vi "DDGImage_.VI"() -> ()   [LabVIEW 2012]
uses:
  <userlib>/atmcd32d.llb/Spool_method typedef.ctl
panel:
  in  "array":i32[](array[numeric])
  out "err string 2":string
  out "强度图 2":i32[][](graph)
  out "err string":string
  out "error out 2":errorcluster
  out "error out":errorcluster
  out "last":i32
  out "first":u32
  out "布尔":bool
  out "强度图":i32[][](graph)
  out "Calculated Kinetic Cycle Time":sgl format="%.2f"
  in  "Frequency (Hz):":dbl format="%.2f"
  in  "Integrate on chip":bool
  in  "Gate step (nsecs)":i32 step=25
  in  "Pulse Width (nsecs)":i32=1000
  in  "Delay (nsecs)":i32 step=25
  in  "Output A Delay (nsecs)":i32 min=0 step=16
  in  "Gain (0-255)":i32 min=0 max=255
  in  "Kinetic Cycle Time":sgl format="%.2f"
  in  "Shut Down":bool
  in  "Start Acquisition":bool
  out "Return  from Get Acquired Data":u32
  out "Detector X Pixels":i32
  out "Return from GetStatus":u32
  out "Return from Start Acquisition":u32
  in  "Number of Kinetics":i32=5
  out "Return from CheckTimings Exposure":u32
  out "Calculated Exposure Value":sgl format="%.2f"
  in  "Exposure Time (secs)":sgl=0.05 format="%.2f"
  out "Return from Initialize":u32
  in  "Trigger":u32(ring) items=["Internal", "External"]
  # "Acquisition Mode: Kinetics\nReadout Mode: Full Image.  Only showing one image of data."
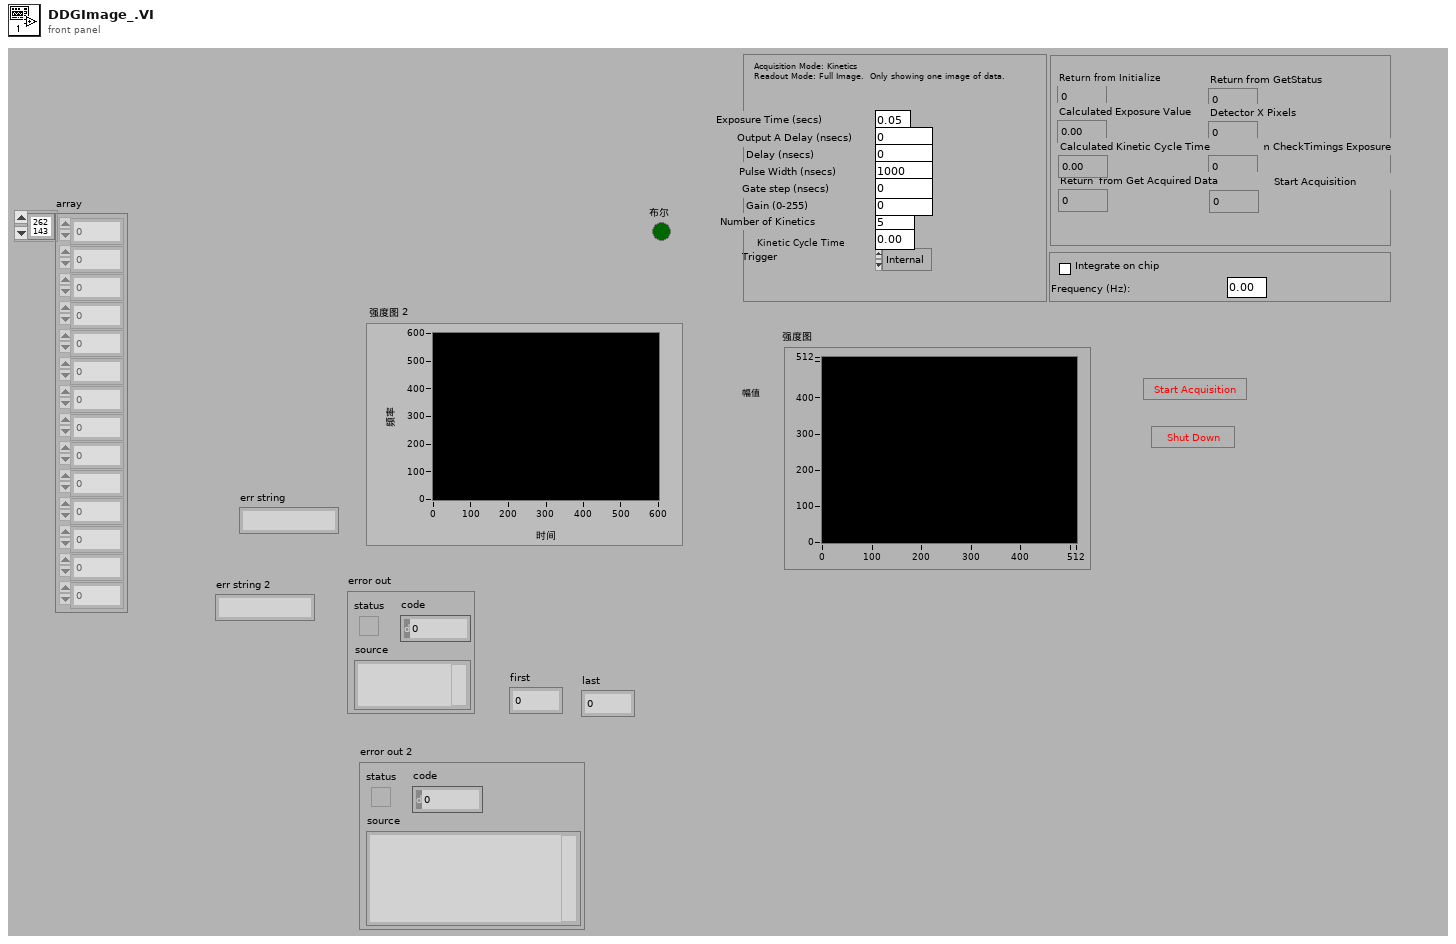
[diagram p1: front panel]
types:
  T1 = typedef "Spool_method typedef.ctl" = enum16{"32-bit", "Depends", "16-bit", "Multiple Directory", "Spool to RAM disk", "16-bit FITS", "SIF", "16-buit TIFF", "Multiple Directory Compressed"}
  T2 = typedef "Error Code Enum typedef.ctl" = enum32{"N/A (0)", "DRV_ERROR_CODES", "DRV_SUCCESS", "DRV_VXDNOTINSTALLED", "DRV_ERROR_SCAN", "DRV_ERROR_CHECK_SUM", "DRV_ERROR_FILELOAD", "DRV_UNKNOWN_FUNC", "DRV_ERROR_VXD_INIT", "DRV_ERROR_ADDRESS", "DRV_ERROR_PAGELOCK", "DRV_ERROR_PAGEUNLOCK", "DRV_ERROR_BOARDTEST", "DRV_ERROR_ACK", "DRV_ERROR_UP_FIFO", "DRV_ERROR_PATTERN", "N/A (16)", "DRV_ACQUISITION_ERRORS", "DRV_ACQ_BUFFER", "DRV_ACQ_DOWNFIFO_FULL", "DRV_PROC_UNKONWN_INSTRUCTION", "DRV_ILLEGAL_OP_CODE", "DRV_KINETIC_TIME_NOT_MET", "DRV_ACCUM_TIME_NOT_MET", "DRV_NO_NEW_DATA", "N/A (25)", "DRV_SPOOLERROR", "N/A (27)", "N/A (28)", "N/A (29)", "N/A (30)", "N/A (31)", "N/A (32)", "DRV_TEMPERATURE_CODES", "DRV_TEMPERATURE_OFF", "DRV_TEMPERATURE_NOT_STABILIZED", "DRV_TEMPERATURE_STABILIZED", "DRV_TEMPERATURE_NOT_REACHED", "DRV_TEMPERATURE_OUT_RANGE", "DRV_TEMPERATURE_NOT_SUPPORTED", "DRV_TEMPERATURE_DRIFT", "N/A (41)", "N/A (42)", "N/A (43)", "N/A (44)", "N/A (45)", "N/A (46)", "N/A (47)", "N/A (48)", "DRV_GENERAL_ERRORS", "DRV_INVALID_AUX", "DRV_COF_NOTLOADED", "DRV_FPGAPROG", "DRV_FLEXERROR", "DRV_GPIBERROR", "N/A (55)", "N/A (56)", "N/A (57)", "N/A (58)", "N/A (59)", "N/A (60)", "N/A (61)", "N/A (62)", "N/A (63)", "DRV_DATATYPE", "DRV_DRIVER_ERRORS", "DRV_P1INVALID", "DRV_P2INVALID", "DRV_P3INVALID", "DRV_P4INVALID", "DRV_INIERROR", "DRV_COFERROR", "DRV_ACQUIRING", "DRV_IDLE", "DRV_TEMPCYCLE", "DRV_NOT_INITIALIZED", "DRV_P5INVALID", "DRV_P6INVALID", "DRV_INVALID_MODE", "DRV_INVALID_FILTER", "DRV_I2CERRORS", "DRV_I2CDEVNOTFOUND", "DRV_I2CTIMEOUT", "DRV_P7INVALID", "N/A (84)", "N/A (85)", "N/A (86)", "N/A (87)", "N/A (88)", "N/A (89)", "DRV_IOCERROR", "DRV_VRMVERSIONERROR"}
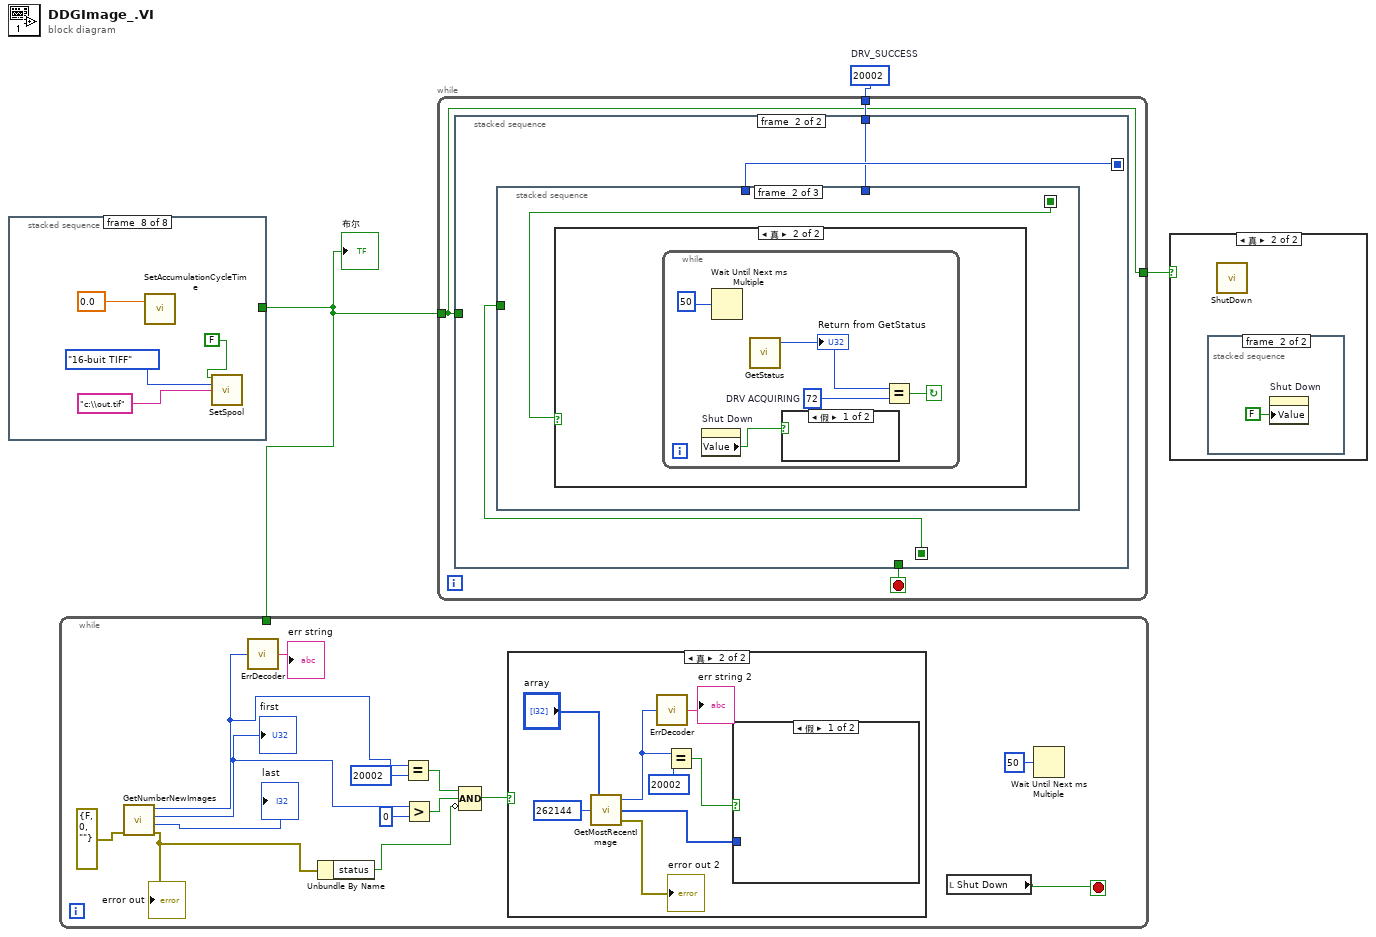
[diagram p0: block diagram]
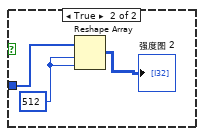
[diagram p3: hidden frame]
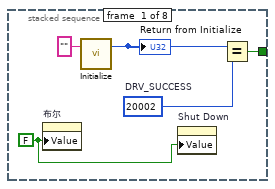
[diagram p4: hidden frame]
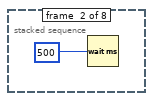
[diagram p5: hidden frame]
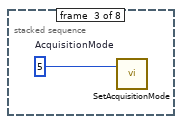
[diagram p6: hidden frame]
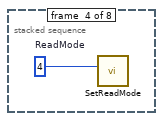
[diagram p7: hidden frame]
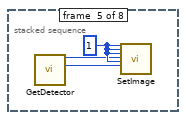
[diagram p8: hidden frame]
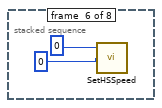
[diagram p9: hidden frame]
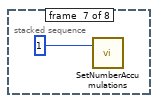
[diagram p10: hidden frame]
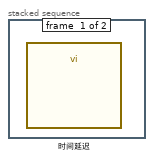
[diagram p12: hidden frame]
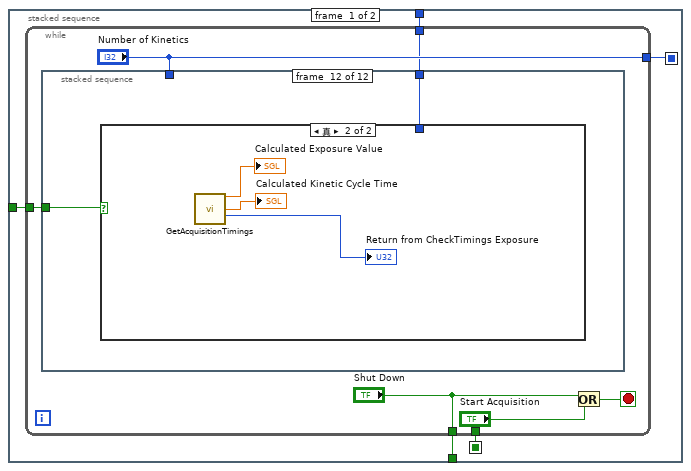
[diagram p13: hidden frame]
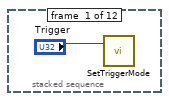
[diagram p14: hidden frame]
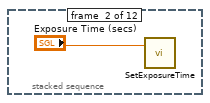
[diagram p15: hidden frame]
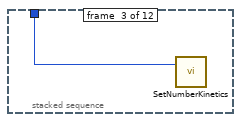
[diagram p16: hidden frame]
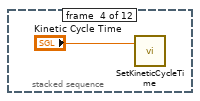
[diagram p17: hidden frame]
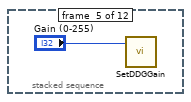
[diagram p18: hidden frame]
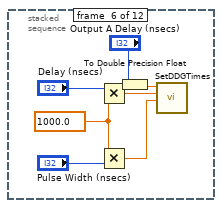
[diagram p19: hidden frame]
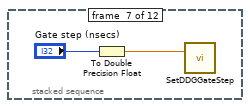
[diagram p20: hidden frame]
diagram:
  w2 = 20002  # DRV_SUCCESS
  n1 = stacked-sequence {
    tunnel: [w5 _ _ _ _ _ _ _] -> w1
    frame #0 {
      w4 = FALSE ("布尔")
      w6 = 20002  # DRV_SUCCESS
      n2 = property on="布尔" class="Bool (严格)"("Value"=w4) -> ()  [unwired: 2 in, 2 out]
      n3 = call <userlib>:"Initialize.vi"("directory (\"\")"="" ("directory (\"\")")) -> ("DLL error code"=w7:u32)  [unwired: 1 in, 1 out]
      "Return from Initialize" <- w7
      n4 = property on="Shut Down" class="Bool (严格)"("Value"=w4) -> ()  [unwired: 2 in, 2 out]
      n5 = Equal?(x=w7, y=w6) -> (x = y?=w5:bool)
    }
    frame #1 {
      n6 = Wait (ms)(milliseconds to wait=u32 500) -> ()  [unwired: 1 out]
    }
    frame #2 {
      w10 = u16 5  # AcquisitionMode
      n7 = call <userlib>:"SetAcquisitionMode.vi"("mode"=w10) -> ()  [unwired: 1 in, 2 out]
    }
    frame #3 {
      w11 = u16 4  # ReadMode
      n8 = call <userlib>:"SetReadMode.vi"("mode"=w11) -> ()  [unwired: 1 in, 2 out]
    }
    frame #4 {
      w14 = 1
      n9 = call <userlib>:"GetDetector.vi"() -> ("ypixels"=w12:i32, "xpixels"=w13:i32)  [unwired: 4 in, 2 out]
      n10 = call <userlib>:"SetImage.vi"("hbin"=w14, "vbin"=w14, "hstart"=w14, "hend"=w13, "vstart"=w14, "vend"=w12) -> ()  [unwired: 20 in, 2 out]
    }
    frame #5 {
      n11 = call <userlib>:"SetHSSpeed.vi"("index"=0, "type"=0) -> ()  [unwired: 2 in, 2 out]
    }
    frame #6 {
      n12 = call <userlib>:"SetNumberAccumulations.vi"("number"=1) -> ()  [unwired: 1 in, 2 out]
    }
    frame #7 {
      n13 = call <userlib>:"SetAccumulationCycleTime.vi"("time"=sgl 0.0) -> ()  [unwired: 1 in, 2 out]
      n14 = call <userlib>:"SetSpool.vi"("active"=FALSE, "method"=Spool_method_typedef."16-buit TIFF", "name"="c:\\out.tif") -> ()  [unwired: 11 in, 2 out]
    }
  }
  "布尔" <- w1
  n15 = while {
    tunnel: w1 -> [_]
    stop <- w24 stop-if-true
    n16 = call <userlib>:"GetNumberNewImages.vi"("error in (no error)"=errorcluster {"status"=FALSE, "code"=0, "source"=""}) -> ("error out"=w32:errorcluster, "last"=→"last":i32, "first"=w30:u32, "DLL error code"=w23:u32)  [unwired: 3 in]
    "first" <- w30
    "error out" <- w32
    n17 = call "ErrDecoder.vi"("err code"=w23) -> ("err string"=→"err string":string)
    n18 = Unbundle By Name(w32) -> ("status"=w26:bool)
    n19 = Equal?(x=w23, y=u32 20002) -> (x = y?=w28:bool)
    n20 = Greater?(x=w30, y=u32 0) -> (0:w27:bool)
    n21 = Compound Arithmetic op=AND(w28, w27, invert w26) -> (w25:bool)
    n22 = case shown="真" w25 {
      frame False {
      }
      frame True {
        n23 = call <userlib>:"GetMostRecentImage.vi"("size"=262144, "array"="array") -> ("error out"=→"error out 2":errorcluster, "array"=w41:i32[], "DLL error code"=w38:u32)  [unwired: 1 in]
        n24 = call "ErrDecoder.vi"("err code"=w38) -> ("err string"=→"err string 2":string)
        n25 = Equal?(x=w38, y=u32 20002) -> (x = y?=w40:bool)
        n26 = case shown="假" w40 {
          tunnel: w41 -> [_ w45]
          frame False {
          }
          frame True {
            w46 = 512 ("维数大小")
            n27 = Reshape Array(w45, w46, w46) -> (→"强度图 2":i32[][])
          }
        }
      }
    }
    n28 = local read "Shut Down"() -> (w24:bool)
    n29 = Wait Until Next ms Multiple(millisecond multiple=u32 50 ("毫秒倍数")) -> ()  [unwired: 1 out]
  }
  n30 = while {
    tunnel: [w47] -> w3
    tunnel: w1 -> [w47]
    tunnel: w2 -> [w48]
    stop <- w49 stop-if-true
    n31 = stacked-sequence {
      seq-local: [w53 _] -> [_ w84]
      seq-local: [w50 _] -> [_ w82]
      tunnel: [w54 _] -> w49
      tunnel: w47 -> [w52 _]
      tunnel: w48 -> [w51 w83]
      frame #0 {
        n32 = while {
          tunnel: ["Shut Down"] -> w54
          tunnel: ["Number of Kinetics"] -> w53
          tunnel: w52 -> [w57]
          tunnel: w51 -> [w56]
          tunnel: ["Start Acquisition"] -> w50
          stop <- w60 stop-if-true
          n33 = stacked-sequence {
            tunnel: "Number of Kinetics" -> [_ _ w63 _ _ _ _ _ _ _ _ _]
            tunnel: w57 -> [_ _ _ _ _ _ _ _ _ _ _ w78]
            tunnel: w56 -> [_ _ _ _ _ _ _ _ _ _ _ w77]
            frame #0 {
              n34 = call <userlib>:"SetTriggerMode.vi"("mode"="Trigger") -> ()  [unwired: 1 in, 2 out]
            }
            frame #1 {
              n35 = call <userlib>:"SetExposureTime.vi"("time"="Exposure Time (secs)") -> ()  [unwired: 1 in, 2 out]
            }
            frame #2 {
              n36 = call <userlib>:"SetNumberKinetics.vi"("number"=w63) -> ()  [unwired: 1 in, 2 out]
            }
            frame #3 {
              n37 = call <userlib>:"SetKineticCycleTime.vi"("time"="Kinetic Cycle Time") -> ()  [unwired: 1 in, 2 out]
            }
            frame #4 {
              n38 = call <userlib>:"SetDDGGain.vi"("gain"="Gain (0-255)") -> ()  [unwired: 1 in, 2 out]
            }
            frame #5 {
              w68 = 1000.0
              n39 = Multiply(x="Delay (nsecs)", y=w68) -> (x*y=w66:dbl)
              n40 = Multiply(x=w68, y="Pulse Width (nsecs)") -> (x*y=w67:dbl)
              n41 = To Double Precision Float(number="Output A Delay (nsecs)") -> (double precision float=w71:dbl)
              n42 = call <userlib>:"SetDDGTimes.vi"("T2"=w67, "T1"=w66, "T0"=w71) -> ()  [unwired: 3 in, 2 out]
            }
            frame #6 {
              n43 = To Double Precision Float(number="Gate step (nsecs)") -> (double precision float=w73:dbl)
              n44 = call <userlib>:"SetDDGGateStep.vi"("step"=w73) -> ()  [unwired: 1 in, 2 out]
            }
            frame #7 {
            }
            frame #8 {
            }
            frame #9 {
              n45 = call <userlib>:"SetDDGIOC.vi"("integrate"="Integrate on chip") -> ()  [unwired: 1 in, 2 out]
            }
            frame #10 {
              n46 = call <userlib>:"SetDDGIOCFrequency.vi"("frequency"="Frequency (Hz):") -> ()  [unwired: 1 in, 2 out]
            }
            frame #11 {
              n47 = case shown="真" w78 {
                tunnel: w77 -> [_ _]
                frame False {
                }
                frame True {
                  n48 = call <userlib>:"GetAcquisitionTimings.vi"() -> ("exposure"=→"Calculated Exposure Value":sgl, "kinetic"=→"Calculated Kinetic Cycle Time":sgl, "DLL error code"=→"Return from CheckTimings Exposure":u32)  [unwired: 11 in, 2 out]
                }
              }
            }
          }
          n49 = Or(x="Shut Down", y="Start Acquisition") -> (x .or. y?=w60:bool)
        }
      }
      frame #1 {
        n50 = stacked-sequence {
          seq-local: [w86 _ _] -> [_ w92 _]
          tunnel: w83 -> [w87 _ _]
          tunnel: w82 -> [w85 _ _]
          tunnel: w84 -> [_ _ w106]
          frame #0 {
            n51 = case shown="真" w85 {
              tunnel: [FALSE w91] -> w86
              tunnel: w87 -> [_ w89]
              frame False {
              }
              frame True {
                n52 = call <userlib>:"StartAcquisition.vi"() -> ("DLL error code"=w90:u32)  [unwired: 2 in, 1 out]
                "Return from Start Acquisition" <- w90
                n53 = Equal?(x=w89, y=w90) -> (x = y?=w91:bool)
              }
            }
          }
          frame #1 {
            n54 = case shown="真" w92 {
              frame False {
              }
              frame True {
                n55 = while {
                  stop <- w96 continue-if-true
                  w95 = u16 72  # DRV ACQUIRING
                  n56 = property on="Shut Down" class="Bool (严格)"() -> ("Value"=w93:bool)  [unwired: 2 in, 2 out]
                  n57 = Wait Until Next ms Multiple(millisecond multiple=u32 50) -> ()  [unwired: 1 out]
                  n58 = call <userlib>:"GetStatus.vi"() -> ("status"=w94:T2)  [unwired: 3 in, 2 out]
                  "Return from GetStatus" <- w94
                  n59 = case shown="假" w93 {
                    frame False {
                    }
                    frame True {
                      n60 = call <userlib>:"AbortAcquisition.vi"() -> ()  [unwired: 2 in, 2 out]
                    }
                  }
                  n61 = Equal?(x=w94, y=w95) -> (x = y?=w96:bool)
                }
              }
            }
          }
          frame #2 {
            n62 = call <userlib>:"GetDetector.vi"() -> ("ypixels"=w99:i32, "xpixels"=w100:i32)  [unwired: 4 in, 2 out]
            "Detector X Pixels" <- w100
            n63 = Multiply(x=w100, y=w99) -> (x*y=w102:i32)
            n64 = Multiply(x=w106, y=w102) -> (x*y=w105:i32)
            n65 = call <userlib>:"GetAcquiredData.vi"("size"=w105) -> ("DLL error code"=→"Return  from Get Acquired Data":u32, "array"=w104:i32[])  [unwired: 2 in, 1 out]
            n66 = Array Subset(array=w104, index=0, length=w102) -> (w101:i32[])
            n67 = Reshape Array(w101, w100, w99) -> (→"强度图":i32[][])
          }
        }
      }
    }
  }
  n68 = case shown="真" w3 {
    frame False {
    }
    frame True {
      n69 = stacked-sequence {
        frame #0 {
          n70 = call "时间延迟"() -> ()  [unwired: 11 in, 1 out]
        }
        frame #1 {
          n71 = property on="Shut Down" class="Bool (严格)"("Value"=FALSE ("Shut Down")) -> ()  [unwired: 2 in, 2 out]
        }
      }
      n72 = call <userlib>:"ShutDown.vi"() -> ()  [unwired: 2 in, 2 out]
    }
  }
